vi "7-29-19 Decreasing.vi"() -> ()   [LabVIEW 2016]
uses:
  <userlib>/Levylab/LV to ITX/LVtoITX.lvclass
  <vilib>/Analysis/NI_AALPro.lvlib
panel:
  out "dG/dt/G Vs temp":cluster{"Data":dbl[], "Data":dbl[]}[](graph)
  out "x/y 2":dbl[](array[numeric])
  out "x/y":dbl[](array[numeric])
  out "dG/dt/G Vs Temp Normalized":cluster{"Data":dbl[], "Data":dbl[]}[](graph)
  out "G Vs Time Fitted":cluster{"Data":dbl[], "Data":dbl[]}[](graph)
  out "Wavenames":string[](array[string])
  out "G Vs Time":cluster{"Data":dbl[], "Data":dbl[]}[](graph)
  out "Data":dbl[][](array[numeric])
  in  "File Path":path=path "G:/My Drive/Data/7-30 Decreasing SA03083.dat"
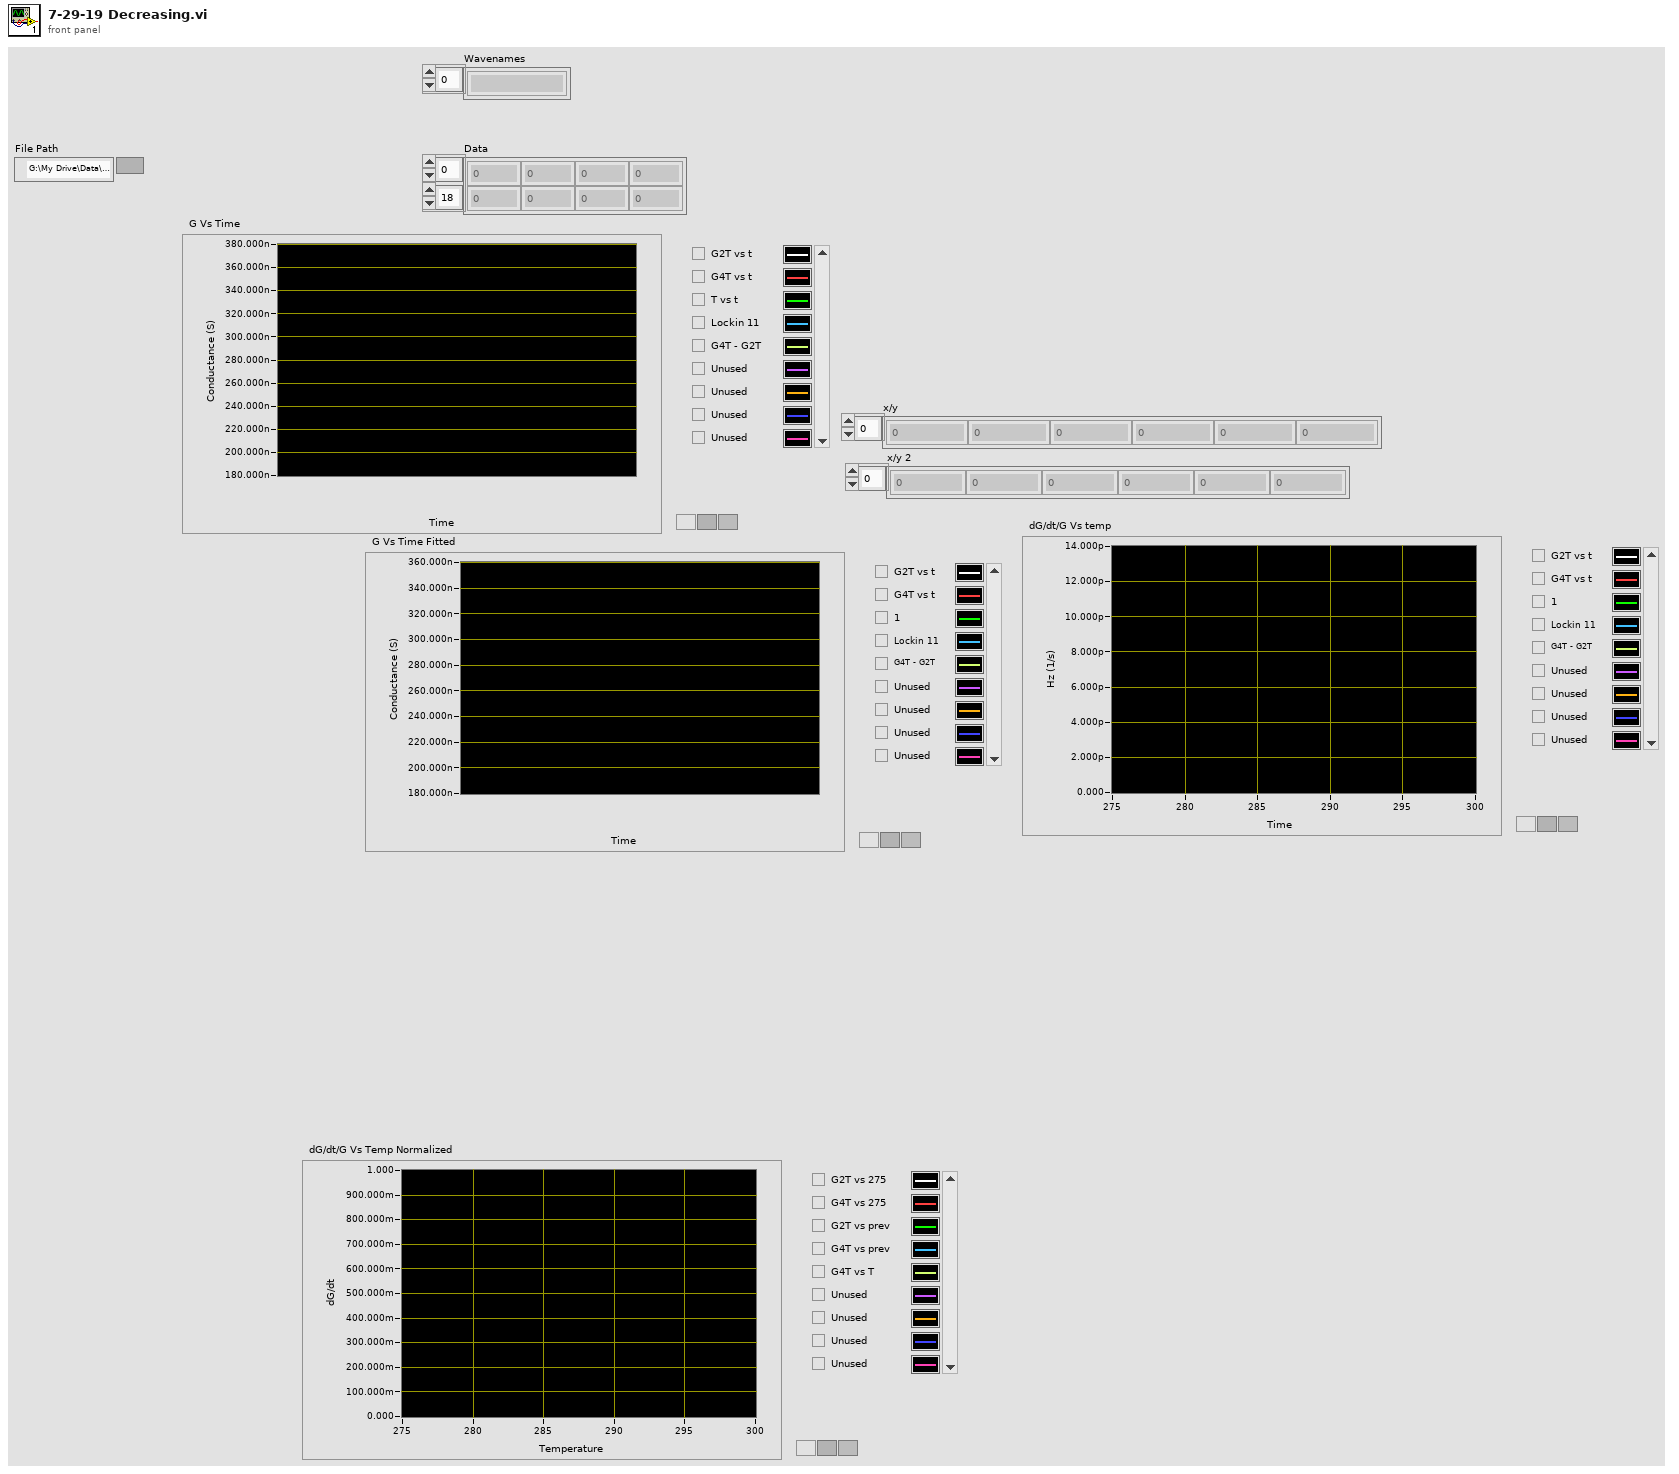
[diagram p1: front panel]
types:
  T1 = cluster{"slope min":dbl, "slope max":dbl, "intercept min":dbl, "intercept max":dbl}
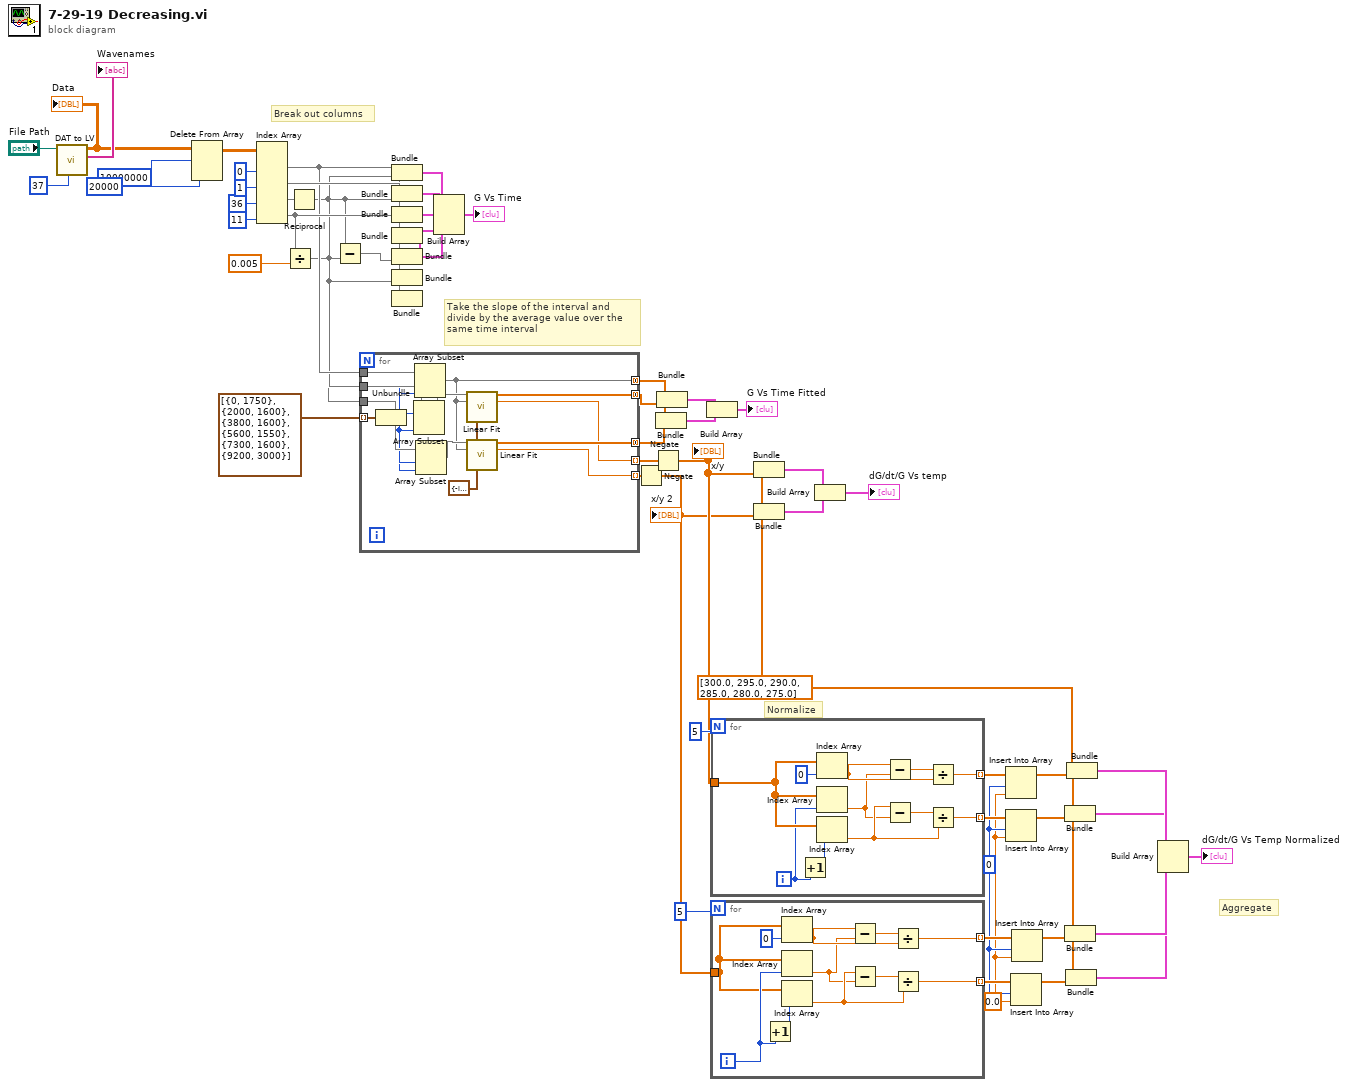
[diagram p0: block diagram]
diagram:
  w4 = dbl[] [300.0, 295.0, 290.0, 285.0, 280.0, 275.0]
  w19 = 0.0 ("new element/subarray")
  w20 = 0 ("index")
  # "Break out columns"
  # "Take the slope of the interval and\ndivide by the average value over the \nsame time interval"
  # "Normalize"
  # "Aggregate"
  n1 = call <userlib>:"DAT to LV.vi"("header length"=37, "File Path"="File Path") -> ("Wavenames"=→"Wavenames":string[], "Data"=w40:dbl[][])  [unwired: 6 in, 2 out]
  "Data" <- w40
  n2 = Delete From Array(array=w40, length=10000000, index (row)=20000) -> (array with subset deleted=w39:dbl[][])  [unwired: 1 in, 1 out]
  n3 = Index Array(array=w39, index (col) #1=0 ("disabled index (col)"), index (col) #2=1 ("index (col)"), index (col) #3=36 ("index (col)"), index (col) #4=11 ("index (col)")) -> (element #1=w34:dbl[], element #2=w53:dbl[], element #3=w46:dbl[], element #4=w36:dbl[])  [unwired: 4 in]
  n4 = Divide(x=w36, y=0.005) -> (x/y=w33:dbl[])
  n5 = Reciprocal(x=w46) -> (1/x=w32:dbl[])
  n6 = Subtract(x=w32, y=w33) -> (x-y=w43:dbl[])
  n7 = for {
    tunnel: cluster{"Index":i32, "Length":i32}[] [{"Index"=0, "Length"=1750}, {"Index"=2000, "Length"=1600}, {"Index"=3800, "Length"=1600}, {"Index"=5600, "Length"=1550}, {"Index"=7300, "Length"=1600}, {"Index"=9200, "Length"=3000}] -> [w71] mode=indexing
    tunnel: w34 -> [w70]
    tunnel: w33 -> [w69]
    tunnel: w32 -> [w68]
    tunnel: [w64] -> w31 mode=concatenating
    tunnel: [w63] -> w30 mode=concatenating
    tunnel: [w60] -> w9 mode=concatenating
    tunnel: [w58] -> w8 mode=indexing
    tunnel: [w59] -> w3 mode=indexing
    w65 = T1 {"slope min"=-inf, "slope max"=inf, "intercept min"=-inf, "intercept max"=inf} ("parameter bounds")
    n8 = Unbundle(w71) -> ("Index"=w67:i32, "Length"=w66:i32)
    n9 = Array Subset(array=w69, index=w67, length=w66) -> (w62:dbl[])
    n10 = Array Subset(array=w70, index=w67, length=w66) -> (w60:dbl[])
    n11 = Array Subset(array=w68, index=w67, length=w66) -> (w61:dbl[])
    n12 = call <vilib>:"Linear Fit.vi"("Y"=w62, "X"=w60, "parameter bounds"=w65) -> ("Best Linear Fit"=w64:dbl[], "slope"=w59:dbl)  [unwired: 8 in, 3 out]
    n13 = call <vilib>:"Linear Fit.vi"("Y"=w61, "X"=w60, "parameter bounds"=w65) -> ("Best Linear Fit"=w63:dbl[], "slope"=w58:dbl)  [unwired: 8 in, 3 out]
  }
  n14 = Bundle("Data"=w34, w33) -> (w38:cluster{"Data":dbl[], dbl[]})  [unwired: 1 in]
  n15 = Bundle("Data"=w34, w32) -> (w37:cluster{"Data":dbl[], dbl[]})  [unwired: 1 in]
  n16 = Bundle("Data"=w34, "Data"=w53) -> (w52:cluster{"Data":dbl[], "Data":dbl[]})  [unwired: 1 in]
  n17 = Bundle("Data"=w34, "Data"=w36) -> (w51:cluster{"Data":dbl[], "Data":dbl[]})  [unwired: 1 in]
  n18 = Bundle("Data"=w34, w43) -> (w44:cluster{"Data":dbl[], dbl[]})  [unwired: 1 in]
  n19 = Bundle("Data"=w53, w33) -> ()  [unwired: 1 in, 1 out]
  n20 = Bundle("Data"=w53, w32) -> ()  [unwired: 1 in, 1 out]
  n21 = Build Array(w38, w37, w52, w51, w44) -> (→"G Vs Time":cluster{"Data":dbl[], "Data":dbl[]}[])
  n22 = Negate(x=w8) -> (-x=w1:dbl[])
  "x/y 2" <- w1
  n23 = Negate(x=w3) -> (-x=w2:dbl[])
  "x/y" <- w2
  n24 = Bundle(w9, "Best Linear Fit"=w30) -> (w29:cluster{dbl[], "Best Linear Fit":dbl[]})  [unwired: 1 in]
  n25 = Bundle(w9, "Best Linear Fit"=w31) -> (w28:cluster{dbl[], "Best Linear Fit":dbl[]})  [unwired: 1 in]
  n26 = Build Array(w28, w29) -> (→"G Vs Time Fitted":cluster{dbl[], "Best Linear Fit":dbl[]}[])
  n27 = for {
    N: 5 -> [_]
    tunnel: w2 -> [w82]
    tunnel: [w76] -> w24 mode=indexing
    tunnel: [w75] -> w23 mode=indexing
    i -> [w80]
    n28 = Increment(x=w80) -> (x+1=w81:i32)
    n29 = Index Array(array=w82, index=0) -> (element=w74:dbl)
    n30 = Index Array(array=w82, index=w80) -> (element=w72:dbl)
    n31 = Index Array(array=w82, index=w81) -> (element=w73:dbl)
    n32 = Subtract(x=w74, y=w72) -> (x-y=w78:dbl)
    n33 = Subtract(x=w73, y=w72) -> (x-y=w77:dbl)
    n34 = Divide(x=w78, y=w74) -> (x/y=w76:dbl)
    n35 = Divide(x=w77, y=w73) -> (x/y=w75:dbl)
  }
  n36 = for {
    N: 5 -> [_]
    tunnel: w1 -> [w88]
    tunnel: [w87] -> w22 mode=indexing
    tunnel: [w86] -> w21 mode=indexing
    i -> [w89]
    n37 = Increment(x=w89) -> (x+1=w90:i32)
    n38 = Index Array(array=w88, index=0) -> (element=w85:dbl)
    n39 = Index Array(array=w88, index=w89) -> (element=w83:dbl)
    n40 = Index Array(array=w88, index=w90) -> (element=w84:dbl)
    n41 = Subtract(x=w85, y=w83) -> (x-y=w92:dbl)
    n42 = Subtract(x=w84, y=w83) -> (x-y=w93:dbl)
    n43 = Divide(x=w92, y=w85) -> (x/y=w87:dbl)
    n44 = Divide(x=w93, y=w84) -> (x/y=w86:dbl)
  }
  n45 = Bundle(w4, w2) -> (w6:cluster{dbl[], dbl[]})  [unwired: 1 in]
  n46 = Bundle(w4, w1) -> (w7:cluster{dbl[], dbl[]})  [unwired: 1 in]
  n47 = Build Array(w6, w7) -> (→"dG/dt/G Vs temp":cluster{dbl[], dbl[]}[])
  n48 = Insert Into Array(array=w24, index=w20, new element=w19) -> (w16:dbl[])
  n49 = Insert Into Array(array=w23, index=w20, new element=w19) -> (w15:dbl[])
  n50 = Insert Into Array(array=w21, index=w20, new element=w19) -> (w17:dbl[])
  n51 = Insert Into Array(array=w22, index=w20, new element=w19) -> (w18:dbl[])
  n52 = Bundle(w4, w15) -> (w12:cluster{dbl[], dbl[]})  [unwired: 1 in]
  n53 = Bundle(w4, w18) -> (w14:cluster{dbl[], dbl[]})  [unwired: 1 in]
  n54 = Bundle(w4, w17) -> (w11:cluster{dbl[], dbl[]})  [unwired: 1 in]
  n55 = Bundle(w4, w16) -> (w13:cluster{dbl[], dbl[]})  [unwired: 1 in]
  n56 = Build Array(w13, w14, w12, w11) -> (→"dG/dt/G Vs Temp Normalized":cluster{dbl[], dbl[]}[])
